vi "Process Data PID 0 control_PD.vi"(6 "output range 2":cluster{"output high":dbl, "output low":dbl}={"output high"=2885.0, "output low"=-2885.0}, 8 "dt IN (s)":dbl=-1.0 format="%.8f", 9 "Froce_mode":bool, 10 "R_force":dbl, 11 "R_force_Ref":dbl) -> (0 "dt OUT (s)":dbl format="%.8f", 3 "Targer Cur R":i16)   [LabVIEW 2019]
uses:
  <vilib>/addons/control/pid/pid.llb/PID (DBL).vi
  <vilib>/addons/control/pid/NI_PID_pid.lvlib
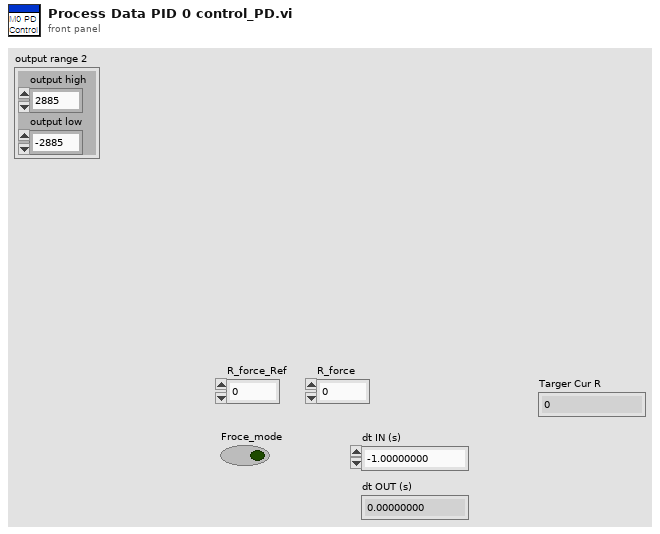
[diagram p1: front panel]
types:
  T1 = cluster{"proportional gain (Kc)":dbl, "integral time (Ti, min)":dbl, "derivative time (Td, min)":dbl}
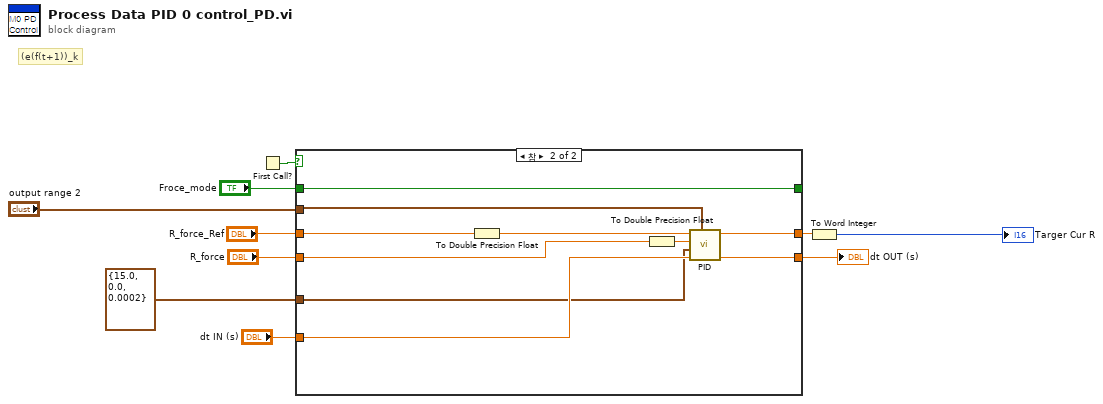
[diagram p0: block diagram]
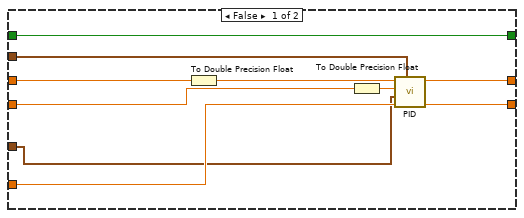
[diagram p2: hidden frame]
diagram:
  # "(e(f(t+1))_k"
  n1 = First Call?() -> (First Call?: T/F=w9:bool)
  n2 = case shown="참" w9 {
    tunnel: [w18 w30] -> w8
    tunnel: "dt IN (s)" -> [w20 w29]
    tunnel: "Froce_mode" -> [w17 w26]
    tunnel: [w19 w22] -> w7
    tunnel: [w17 w26] -> _
    tunnel: "R_force_Ref" -> [w14 w24]
    tunnel: "R_force" -> [w13 w25]
    tunnel: "output range 2" -> [w12 w21]
    tunnel: T1 {"proportional gain (Kc)"=15.0, "integral time (Ti, min)"=0.0, "derivative time (Td, min)"=0.0002} ("PID gains") -> [w11 w23]
    frame False {
      n3 = To Double Precision Float(number=w14) -> (double precision float=w15:dbl)
      n4 = To Double Precision Float(number=w13) -> (double precision float=w16:dbl)
      n5 = call-poly <vilib>:"PID.vi"("output range"=w12, "dt (s)"=w20, "PID gains"=w11, "process variable"=w16, "setpoint"=w15) -> ("dt out (s)"=w18:dbl, "output"=w19:dbl)  [unwired: 5 in]
    }
    frame True {
      n6 = To Double Precision Float(number=w24) -> (double precision float=w27:dbl)
      n7 = To Double Precision Float(number=w25) -> (double precision float=w28:dbl)
      n8 = call-poly <vilib>:"PID.vi"("output range"=w21, "dt (s)"=w29, "PID gains"=w23, "process variable"=w28, "setpoint"=w27) -> ("dt out (s)"=w30:dbl, "output"=w22:dbl)  [unwired: 5 in]
    }
  }
  "dt OUT (s)" <- w8
  n9 = To Word Integer(number=w7) -> (16bit integer=→"Targer Cur R":i16)
